vi "determineSlewFlagValue.vi"(8 "error in (no error)":errorcluster, 10 "SlewFlag":bool, 11 "FAILC in":refnum<class "FAILC.lvclass">) -> (0 "error out":errorcluster, 2 "FlagValue":u8, 3 "FAILC out":refnum<class "FAILC.lvclass">)   [LabVIEW 2016, in "RTFAILC.lvlib" / "FAILC.lvclass"]
uses:
  FAILC.lvclass
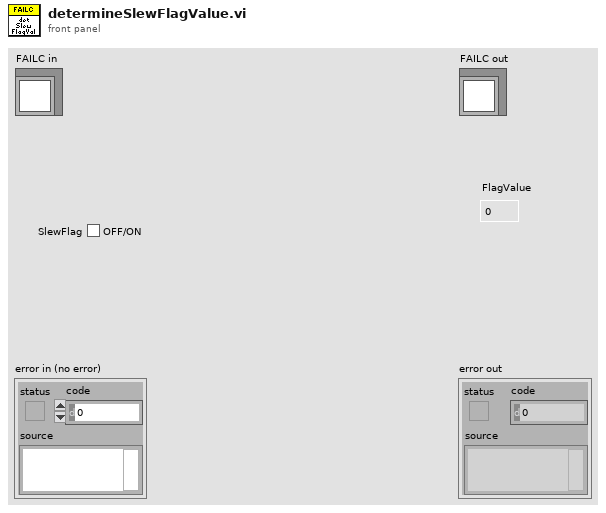
[diagram p1: front panel]
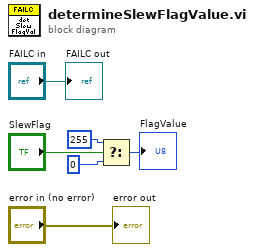
[diagram p0: block diagram]
diagram:
  n1 = Select(t=u8 255, s="SlewFlag", f=u8 0) -> (s? t:f=→"FlagValue":u8)
  "error out" <- "error in (no error)"
  "FAILC out" <- "FAILC in"
